vi "Select and Enable Component.vi"(7 "Disable Others?":bool, 8 "error in (no error)":errorcluster, 10 "Component":string, 11 "Camera in":refnum<class "Camera.lvclass">) -> (0 "error out":errorcluster, 3 "Camera":refnum<class "Camera.lvclass">)   [LabVIEW 2020, in "Camera.lvclass"]
uses:
  Camera.lvclass
  Camera.lvclass/Camera.ctl
  bin/gindustrialcam_32-1.dll
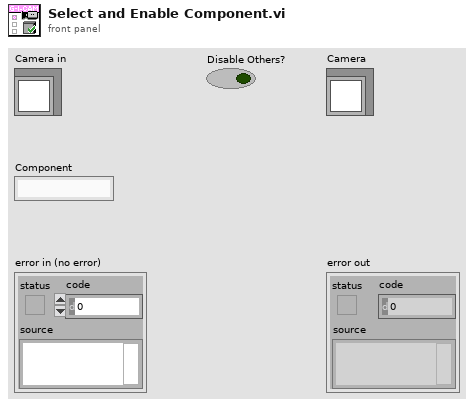
[diagram p1: front panel]
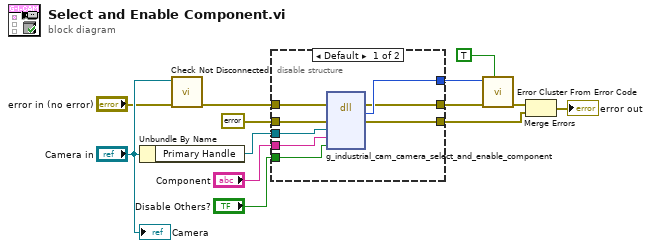
[diagram p0: block diagram]
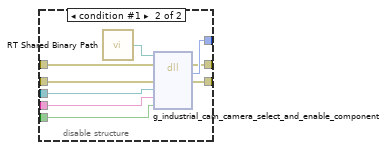
[diagram p2: hidden frame]
diagram:
  n1 = Unbundle By Name("Camera in") -> ("Primary Handle"=w8:refnum<data-value>)
  n2 = call "Check Not Disconnected.vi"("error in (no error)"="error in (no error)", "Camera in"="Camera in") -> ("error out"=w9:errorcluster)  [unwired: 9 in]
  n3 = disable-structure shown="Default" {
    disable-tunnel: "Disable Others?" -> [w21 w30]
    disable-tunnel: w9 -> [w20 w29]
    disable-tunnel: w8 -> [w19 w28]
    disable-tunnel: errorcluster {"status"=FALSE, "code"=0, "source"=""} ("error constant") -> [w18 w27]
    disable-tunnel: [w17 w26] -> w5
    disable-tunnel: [w16 w25] -> w3
    disable-tunnel: [w15 w24] -> w2
    disable-tunnel: "Component" -> [w14 w23]
    frame condition #0 (active) {
      n4 = dll-call lib="C:/serenial/lib/g-industrial-camera/LabVIEW/g_industrial_cam/bin/gindustrialcam_*-1.*" fn="g_industrial_cam_camera_select_and_enable_component"(error in=w20, "err"=w18, "edvr"=w19, "component"=w14, "disable_others"=w21) -> (error out=w15:errorcluster, "Mg_Error"=w16:i32, "err"=w17:errorcluster)  [unwired: 5 in, 1 out]
    }
    frame condition #1 {
      n5 = call "RT Shared Binary Path.vi"() -> ("Path"=w22:path)
      n6 = dll-call lib="C:/serenial/lib/g-industrial-camera/LabVIEW/g_industrial_cam/bin/gindustrialcam_*-1.*" fn="g_industrial_cam_camera_select_and_enable_component"(path in=w22, error in=w29, "err"=w27, "edvr"=w28, "component"=w23, "disable_others"=w30) -> (error out=w24:errorcluster, "Mg_Error"=w25:i32, "err"=w26:errorcluster)  [unwired: 4 in, 1 out]
    }
  }
  n7 = call <vilib>:"Error Cluster From Error Code.vi"("show call chain? (False)"=TRUE, "error in (no error)"=w2, "error code (0)"=w3) -> ("error out"=w4:errorcluster)  [unwired: 6 in]
  n8 = Merge Errors(w4, w5) -> (→"error out":errorcluster)
  "Camera" <- "Camera in"
